vi "Read.vi"(8 "error in":errorcluster, 11 "Chiller Cluster - 1 Channel.lvclass":refnum<class "Device Cluster - 1 Channel.lvclass">) -> (0 "error out":errorcluster, 3 "output cluster":refnum<class "Device Cluster - 1 Channel.lvclass">)   [LabVIEW 2023, in "Device Cluster - 1 Channel.lvclass"]
uses:
  Device Cluster - 1 Channel.lvclass
  Device Cluster - 1 Channel.lvclass/Device Cluster - 1 Channel.ctl
  9c8d422d-920d-4f62-ba29-e6a76558d5ae.vi
  9c8d422d-920d-4f62-ba29-e6a76558d5ae.vi/c28b0ead-42ad-4072-80a2-aca7f2bd7ce3.vi
  9c8d422d-920d-4f62-ba29-e6a76558d5ae.vi/219d0231-d98b-4193-b5cc-84f90e3c9091.vi
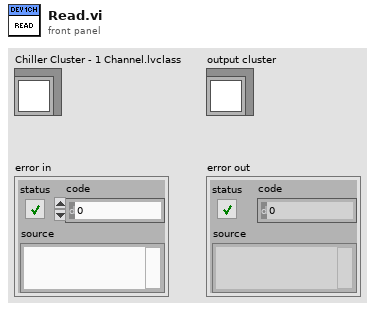
[diagram p1: front panel]
types:
  T1 = cluster{"Voltage.ch01.SP":dbl, "Current.ch01.SP":dbl}
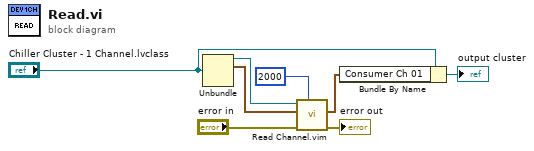
[diagram p0: block diagram]
diagram:
  n1 = Unbundle("Chiller Cluster - 1 Channel.lvclass") -> (w6:refnum<k21>, w5:T1)  [unwired: 2 out]
  n2 = call "Read Channel.vim"("Timeout (ms)"=2000, "error in"="error in", "Data in"=w5, "ADAS HIL Channel in"=w6) -> ("error out"=→"error out":errorcluster, "Data out"=w1:T1)  [unwired: 4 in, 2 out]
  n3 = Bundle By Name(cluster="Chiller Cluster - 1 Channel.lvclass", "Consumer Ch 01"=w1) -> (→"output cluster":refnum<class "Device Cluster - 1 Channel.lvclass">)
